vi "Write Numeric Text Props.vi"(8 "error in":errorcluster, 10 "Numeric Text Props":T1, 11 "Control in":refnum<vi>) -> (0 "error out":errorcluster, 3 "Control":refnum<vi>)   [LabVIEW 2020, in "VolatusGUIEditorCore.lvlib"]
uses:
  VolatusGUIEditorCore.lvlib
  Numeric Text Props.ctl
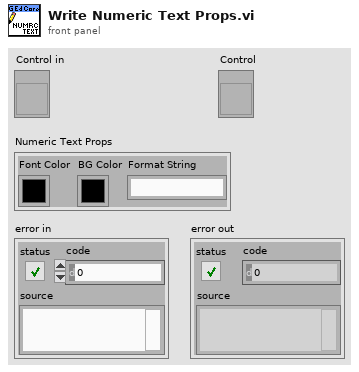
[diagram p1: front panel]
types:
  T1 = typedef "VolatusGUIEditorCore.lvlib/Numeric Text Props.ctl" = cluster{"Font Color":u32, "BG Color":u32, "Format String":string}
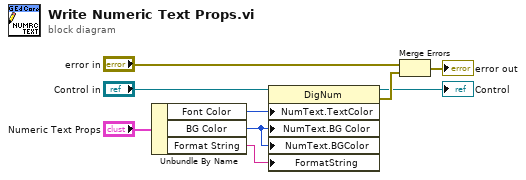
[diagram p0: block diagram]
diagram:
  n1 = Unbundle By Name("Numeric Text Props") -> ("Font Color"=w5:u32, "BG Color"=w4:u32, "Format String"=w3:string)
  n2 = property class="DigNum"(reference="Control in", "NumText.TextColor"=w5, "NumText.BG Color"=w4, "NumText.BGColor"=w4, "FormatString"=w3) -> (reference out=→"Control":refnum<vi>, error out=w9:errorcluster)  [unwired: 1 in]
  n3 = Merge Errors("error in", w9) -> (→"error out":errorcluster)
